vi "AeroQuadLauncher.vi"   [LabVIEW 2009]
types:
  T1 = enum32{"Invalid", "Standard", "Closed", "Hidden", "Minimized", "Maximized"}
  T2 = enum32{"invalid app kind", "Development System", "Run Time System", "Student Edition", "Embedded LabVIEW", "Evaluation", "Custom"}
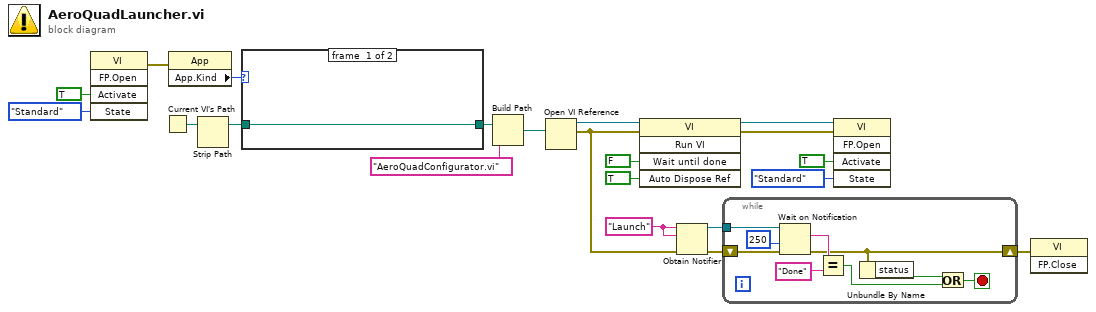
[diagram p0: block diagram]
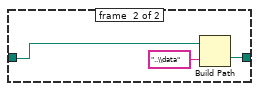
[diagram p2: hidden frame]
diagram:
  w17 = "Launch" ("name (unnamed)")
  n1 = invoke class="VI" method="FP.Open"("Activate"=TRUE ("Activate?"), "State"=T1."Standard") -> (error out=w2:errorcluster)  [unwired: 3 in, 4 out]
  n2 = Current VI's Path() -> (path=w21:path)
  n3 = property class="App"(error in=w2) -> ("App.Kind"=w8:T2)  [unwired: 1 in, 2 out]
  n4 = Strip Path(path=w21) -> (stripped path=w9:path)  [unwired: 1 out]
  n5 = case shown="\"Run Time System\", Default" w8 {
    tunnel: w9 -> [w22 w24]
    tunnel: [w22 w25] -> w7
    frame #0 {
    }
    frame #1 {
      n6 = Build Path(base path=w24, name or relative path="..\\data") -> (appended path=w25:path)
    }
  }
  n7 = Build Path(base path=w7, name or relative path="AeroQuadConfigurator.vi") -> (appended path=w11:path)
  n8 = Open VI Reference(vi path=w11) -> (vi reference=w20:refnum<vi>, error out=w1:errorcluster)  [unwired: 5 in]
  n9 = invoke class="VI" method="Run VI"(reference=w20, error in=w1, "Wait until done"=FALSE ("Wait Until Done"), "Auto Dispose Ref"=TRUE ("Auto Dispose Reference")) -> (reference out=w6:refnum<vi>, error out=w3:errorcluster)  [unwired: 1 in, 3 out]
  n10 = Obtain Notifier(name (unnamed)=w17, notification data type=w17, error in (no error)=w1) -> (notifier out=w15:refnum<notifier>, error out=w16:errorcluster)  [unwired: 1 in, 1 out]
  n11 = while {
    shift-right: [w28] -> w14
    shift-left: w16 -> [w34]
    tunnel: w15 -> [w33]
    stop <- w26 stop-if-true
    n12 = Wait on Notification(notifier=w33, timeout in ms (-1)=250, error in (no error)=w34) -> (notification=w31:string, error out=w28:errorcluster)  [unwired: 1 in, 2 out]
    n13 = Equal?(x=w31, y="Done") -> (x = y?=w29:bool)
    n14 = Unbundle By Name(w28) -> ("status"=w27:bool)
    n15 = Or(x=w27, y=w29) -> (x .or. y?=w26:bool)
  }
  n16 = invoke class="VI" method="FP.Open"(reference=w6, error in=w3, "Activate"=TRUE ("Activate?"), "State"=T1."Standard") -> ()  [unwired: 1 in, 5 out]
  n17 = invoke class="VI" method="FP.Close"(error in=w14) -> ()  [unwired: 2 in, 3 out]
